vi "Piccolo Raw Data Decoding.vi"(8 "TDC U32":u32, 11 "Photon U32":u32) -> (0 "TDC U32":u32, 1 "Y":u8, 2 "X":u8, 3 "TDC Bin":u16)   [LabVIEW 2021, in "Piccolo.lvlib"]
uses:
  Piccolo.lvlib
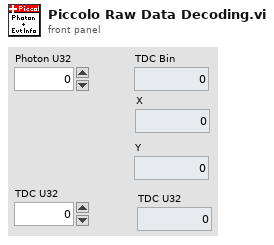
[diagram p1: front panel]
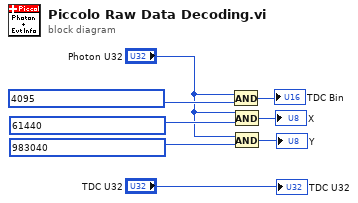
[diagram p0: block diagram]
diagram:
  n1 = And(x="Photon U32", y=u32 4095) -> (x .and. y?=→"TDC Bin":u32)
  n2 = And(x="Photon U32", y=u32 61440) -> (x .and. y?=→"X":u32)
  n3 = And(x="Photon U32", y=u32 983040) -> (x .and. y?=→"Y":u32)
  "TDC U32" <- "TDC U32"
